vi "Add dllspec To Functions Prototypes.vi"(8 "Error In":errorcluster, 10 "dllspec token":string="EXAMPLE_DLL", 11 "input string":string="long lubo();\nint something else();\n\nvoid ugo(int a = 0);\n") -> (0 "Error Out":errorcluster, 3 "String":string)   [LabVIEW 2014]
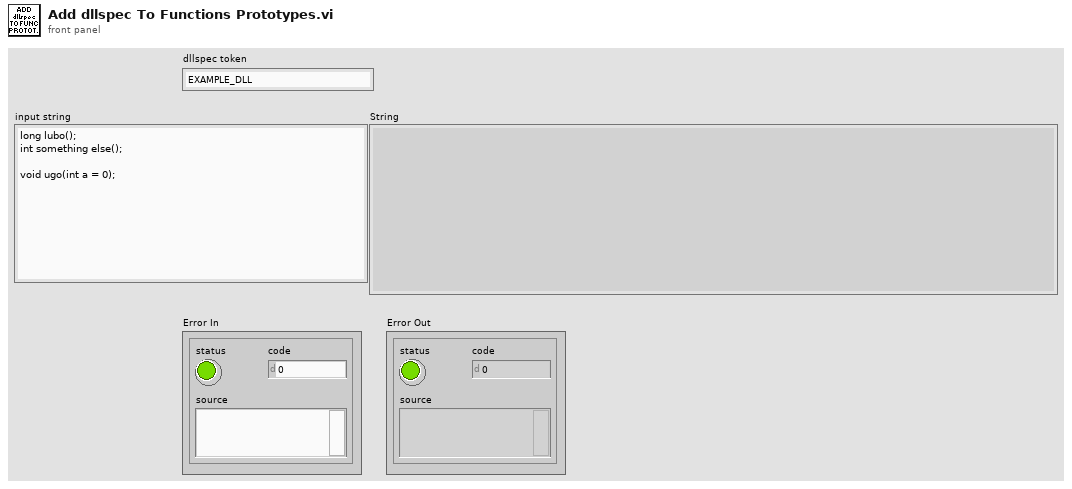
[diagram p1: front panel]
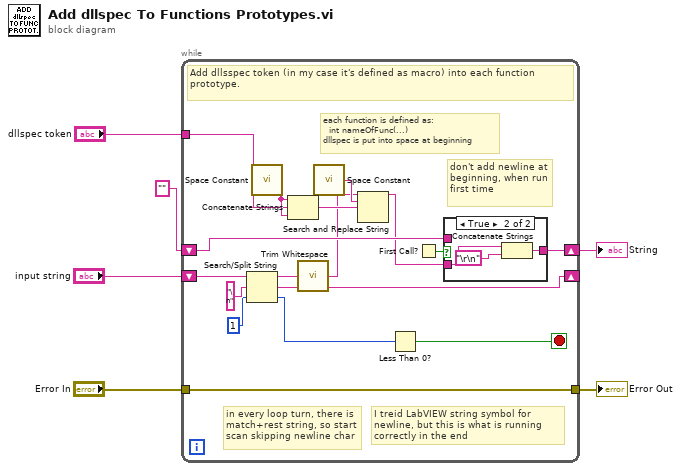
[diagram p0: block diagram]
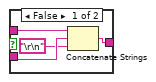
[diagram p2: hidden frame]
diagram:
  n1 = while {
    tunnel: "Error In" -> [w17]
    shift-right: [w23] -> w2
    shift-left: "" -> [w22]
    shift-right: [w20] -> _
    shift-left: "input string" -> [w21]
    tunnel: [w17] -> w3
    tunnel: "dllspec token" -> [w11]
    stop <- w19 stop-if-true
    # "in every loop turn, there is match+rest string, so start scan skipping newline char"
    # "don't add newline at beginning, when run first time"
    # "I treid LabVIEW string symbol for newline, but this is what is running correctly in the end"
    # "each function is defined as:\n  int nameOfFunc(...)\ndllspec is put into space at beginning"
    # "Add dllsspec token (in my case it's defined as macro) into each function prototype."
    n2 = Search/Split String(string=w21, search string/char (-)="\n", offset (0)=1) -> (substring before match=w9:string, match + rest of string=w20:string, offset of match=w18:i32)
    n3 = call <vilib>:"Space Constant.vi"() -> ("String"=w14:string)
    n4 = Concatenate Strings(w14, w11, w14) -> (w13:string)
    n5 = call <vilib>:"Trim Whitespace.vi"("string"=w9) -> ("trimmed string"=w8:string)  [unwired: 1 in]
    n6 = call <vilib>:"Space Constant.vi"() -> ("String"=w12:string)
    n7 = Search and Replace String(input string=w8, search string=w12, replace string=w13) -> (result string=w10:string)  [unwired: 5 in, 3 out]
    n8 = Less Than 0?(x=w18) -> (x < 0?=w19:bool)
    n9 = First Call?() -> (First Call?: T/F=w15:bool)
    n10 = case shown="True" w15 {
      tunnel: [w27 w29] -> w23
      tunnel: w22 -> [w26 _]
      tunnel: w10 -> [w25 w30]
      frame False {
        n11 = Concatenate Strings(w26, w25, "\r\n") -> (w27:string)
      }
      frame True {
        n12 = Concatenate Strings(w30, "\r\n") -> (w29:string)
      }
    }
  }
  "Error Out" <- w3
  "String" <- w2
